vi "positionTest.vi"() -> (0 "BackRight":dbl, 1 "BackLeft":dbl, 2 "FrontRight":dbl, 3 "FrontLeft":dbl)   [LabVIEW 2011]
panel:
  in  "button4":bool
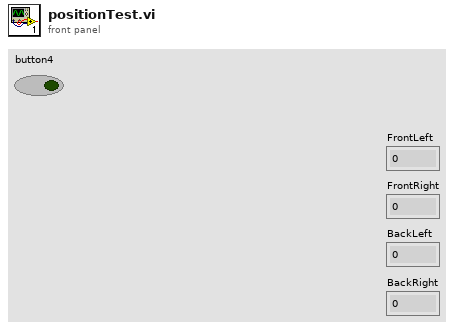
[diagram p1: front panel]
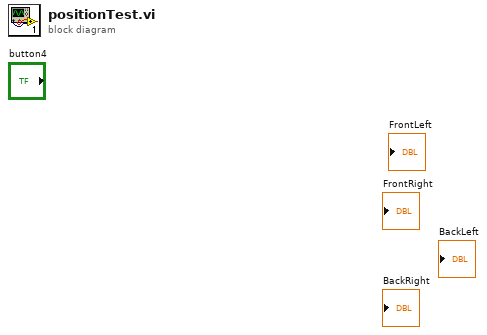
[diagram p0: block diagram]
diagram:
